vi "Get Size.vi"(8 "1D Array":u64[](array[numeric]), 11 "2D Array":u64[][](array[numeric])) -> (0 "1D Size":i32, 1 "RowColSizeArr":i32[](array[numeric]), 2 "colSize":i32, 3 "row Size":i32)   [LabVIEW 2023]
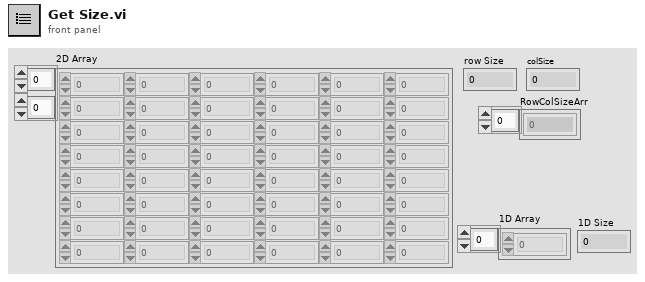
[diagram p1: front panel]
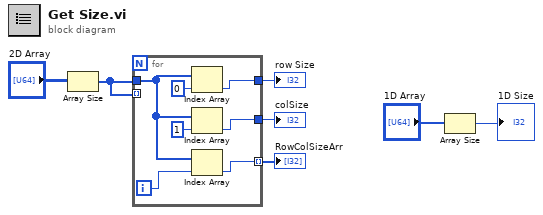
[diagram p0: block diagram]
diagram:
  n1 = Array Size(array="2D Array") -> (size(s)=w4:i32[])
  n2 = for {
    tunnel: w4 -> [w9]
    tunnel: w4 -> [_] mode=indexing
    tunnel: [w14] -> w3
    tunnel: [w11] -> w2
    tunnel: [w8] -> w1 mode=indexing
    i -> [w10]
    n3 = Index Array(array=w9, index=0) -> (element=w14:i32)
    n4 = Index Array(array=w9, index=1) -> (element=w11:i32)
    n5 = Index Array(array=w9, index=w10) -> (element=w8:i32)
  }
  "row Size" <- w3
  "colSize" <- w2
  "RowColSizeArr" <- w1
  n6 = Array Size(array="1D Array") -> (size(s)=→"1D Size":i32)
